vi "Make Section Images SubVI.vi"(6 "Image width":i32, 7 "Image in":T1, 8 "error in (no error)":errorcluster, 9 "Footer Info":T2, 10 "Main Body Info":T2, 11 "Header Info":T2) -> (0 "error out":errorcluster, 1 "Footer Image":T1(plugin-control), 2 "Main Body Image":T1(plugin-control), 3 "Header Image":T1(plugin-control))   [LabVIEW 2018, in "Image Management.lvlib"]
uses:
  Image Management.lvlib
  receipt parsing/Section Info--cluster.ctl
  <vilib>/vision/Image Controls.llb/IMAQ Image.ctl
  <vilib>/vision/NI_Vision_Development_Module.lvlib
  receipt parsing/Receipt Parsing.lvlib
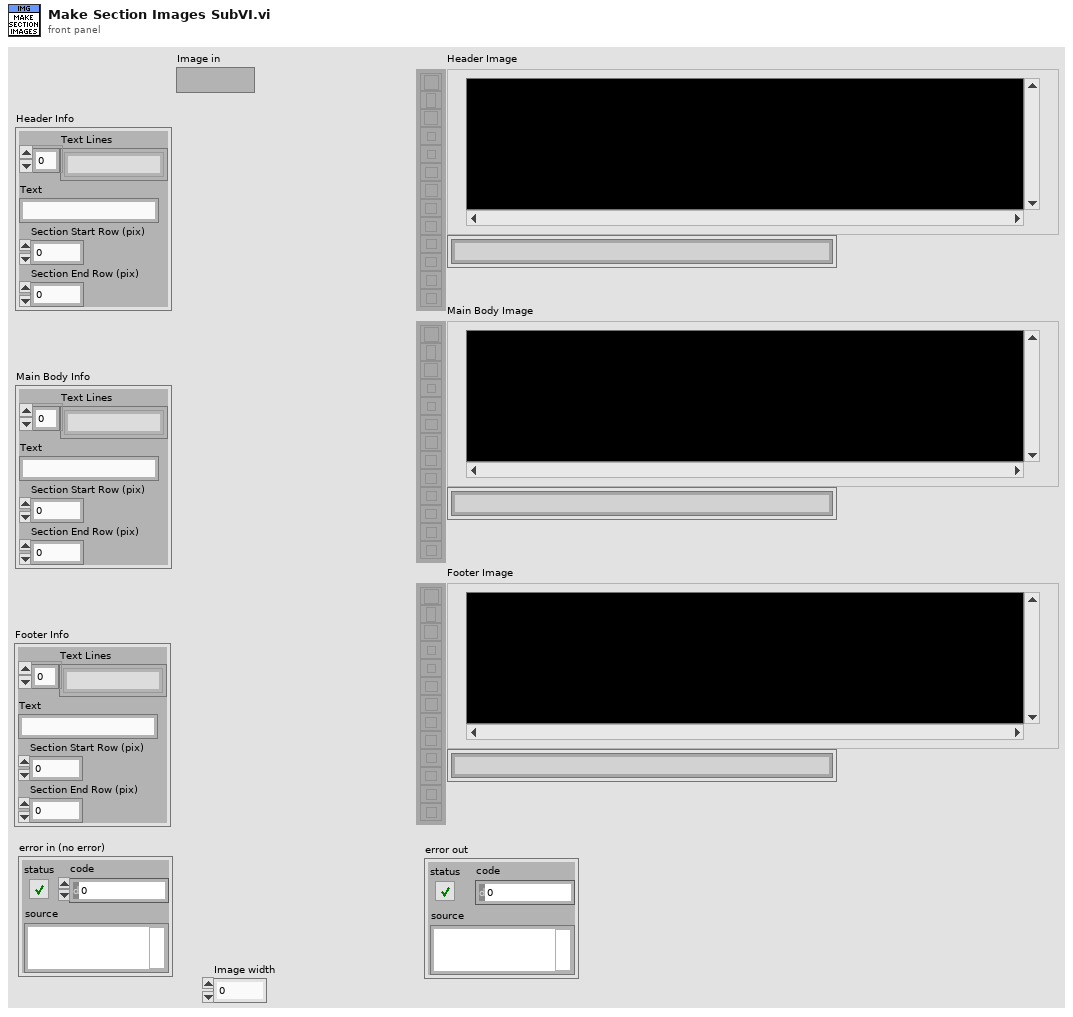
[diagram p1: front panel]
types:
  T1 = typedef "IMAQ Image.ctl" = refnum<image>
  T2 = typedef "Receipt Parsing.lvlib/Section Info--cluster.ctl" = cluster{"Text Lines":string[], "Text":string, "Section Start Row (pix)":i32, "Section End Row (pix)":i32}
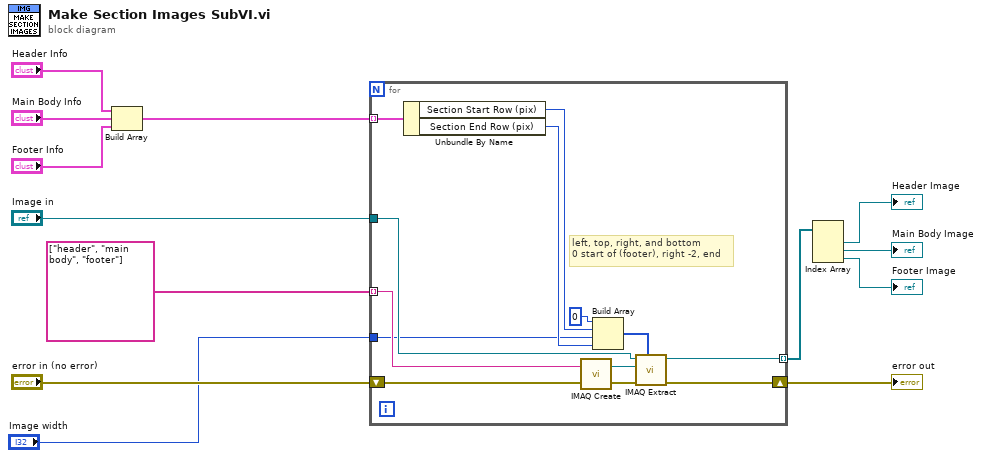
[diagram p0: block diagram]
diagram:
  n1 = Build Array("Header Info", "Main Body Info", "Footer Info") -> (w8:T2[])
  n2 = for {
    shift-right: [w26] -> w13
    shift-left: "error in (no error)" -> [w25]
    tunnel: "Image in" -> [w23]
    tunnel: [w24] -> w11 mode=indexing
    tunnel: string[] ["header", "main body", "footer"] -> [w16] mode=indexing
    tunnel: w8 -> [w15] mode=indexing
    tunnel: "Image width" -> [w14]
    # "left, top, right, and bottom \n0 start of (footer), right -2, end"
    n3 = Unbundle By Name(w15) -> ("Section Start Row (pix)"=w18:i32, "Section End Row (pix)"=w17:i32)
    n4 = call "IMAQ Create"("Image Name"=w16, "error in (no error)"=w25) -> ("New Image"=w22:T1, "error out"=w21:errorcluster)  [unwired: 3 in]
    n5 = Build Array(0 ("element"), w18, w14, w17) -> (w20:i32[])
    n6 = call "IMAQ Extract"("Optional Rectangle"=w20, "error in (no error)"=w21, "Image Dst"=w22, "Image Src"=w23) -> ("error out"=w26:errorcluster, "Image Dst Out"=w24:T1)  [unwired: 6 in]
  }
  "error out" <- w13
  n7 = Index Array(array=w11) -> (element #1=→"Header Image":T1, element #2=→"Main Body Image":T1, element #3=→"Footer Image":T1)  [unwired: 3 in]
